vi "Close.vi"(8 "error in (no error)":errorcluster, 11 "uService Template in":refnum<class "TCP Writer.lvclass">) -> (0 "error out":errorcluster, 3 "uService Template out":refnum<class "TCP Writer.lvclass">)   [LabVIEW 2026, in "TALOS.lvlib" / "TCP Writer.lvlib" / "TCP Writer.lvclass"]
uses:
  TCP Writer.lvclass
  Father of all uServices/Father of all uServices/Father of all uServices.lvclass
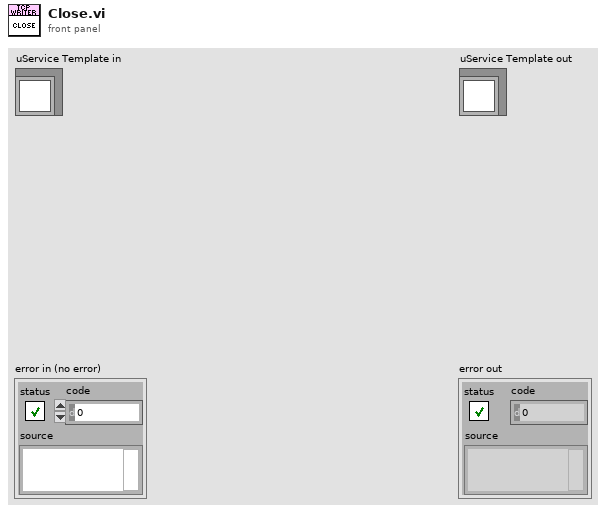
[diagram p1: front panel]
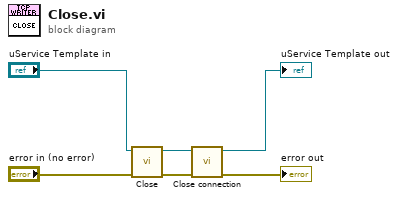
[diagram p0: block diagram]
diagram:
  n1 = call-parent "Close.vi"("error in (no error)"="error in (no error)", "uService Template in"="uService Template in") -> ("error out"=w6:errorcluster, "uService Template out"=w3:refnum<class "TCP Writer.lvclass">)  [unwired: 8 in]
  n2 = call-dynamic "Close connection.vi"("error in (no error)"=w6, "TCP Writer in"=w3) -> ("error out"=→"error out":errorcluster, "TCP Writer out"=→"uService Template out":refnum<class "TCP Writer.lvclass">)  [unwired: 8 in]
